vi "ErrorState.vi"(8 "error in (no error)":errorcluster, 11 "Caller in":refnum<class "Caller.lvclass">) -> (0 "error out":errorcluster, 3 "Caller out":refnum<class "Caller.lvclass">)   [LabVIEW 2020, in "Caller.lvlib" / "Caller.lvclass"]
uses:
  Caller.lvclass
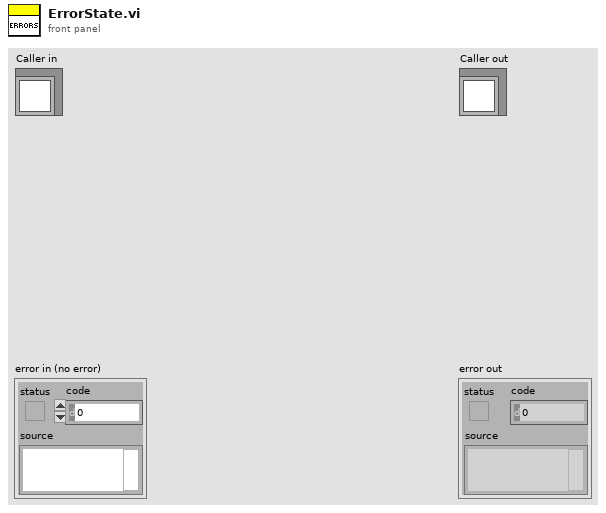
[diagram p1: front panel]
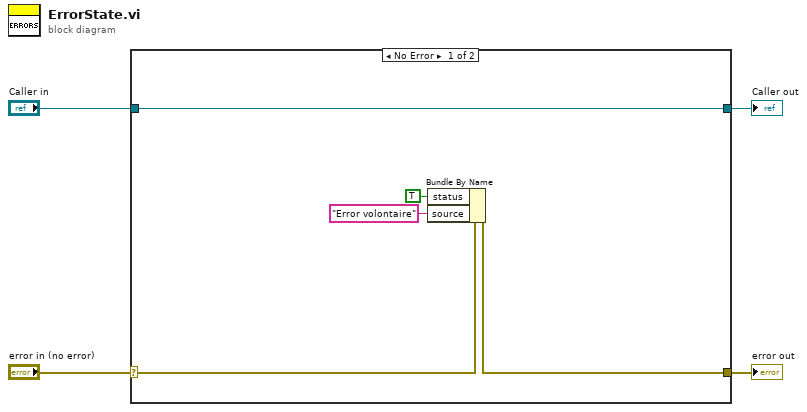
[diagram p0: block diagram]
diagram:
  n1 = case shown="No Error" "error in (no error)" {
    selector: "error in (no error)" -> [w8 w11]
    tunnel: [w7 w11] -> w3
    tunnel: [w9 w10] -> w1
    tunnel: "Caller in" -> [w9 w10]
    frame No Error {
      n2 = Bundle By Name(cluster=w8, "status"=TRUE, "source"="Error volontaire") -> (w7:errorcluster)
    }
    frame Error {
    }
  }
  "error out" <- w3
  "Caller out" <- w1
